vi "Input Panel Resize.vi"(8 "NewBnds":T1, 11 "Entry Panel in":refnum<vi>[](array[refnum])) -> (3 "Entry Panel out":refnum<vi>[](array[refnum]))   [LabVIEW 2015, in "CallVIStep.lvclass"]
uses:
  CallVIStep.lvclass
  <vilib>/Utility/miscctls.llb/LVRectTypeDef.ctl
  <vilib>/Utility/miscctls.llb/LVPositionTypeDef.ctl
  <vilib>/Utility/miscctls.llb/LVBoundsTypeDef.ctl
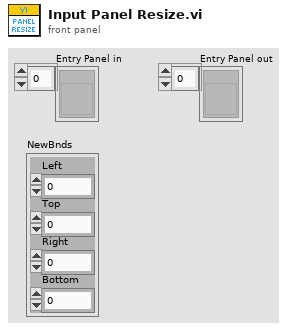
[diagram p1: front panel]
types:
  T1 = typedef "LVRectTypeDef.ctl" = cluster{"Left":i16, "Top":i16, "Right":i16, "Bottom":i16}
  T2 = typedef "LVBoundsTypeDef.ctl" = cluster{"Width":u32, "Height":u32}
  T3 = typedef "LVPositionTypeDef.ctl" = cluster{"Left":i32, "Top":i32}
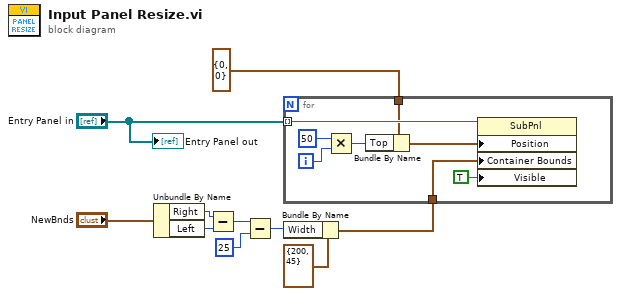
[diagram p0: block diagram]
diagram:
  n1 = Unbundle By Name("NewBnds") -> ("Right"=w7:i16, "Left"=w6:i16)
  n2 = Subtract(x=w7, y=w6) -> (x-y=w8:i16)
  n3 = Subtract(x=w8, y=i16 25) -> (x-y=w10:i16)
  n4 = Bundle By Name(cluster=T2 {"Width"=200, "Height"=45} ("Container Bounds"), "Width"=w10) -> (w2:T2)
  n5 = for {
    tunnel: "Entry Panel in" -> [w18] mode=indexing
    tunnel: T3 {"Left"=0, "Top"=0} ("Position") -> [w17]
    tunnel: w2 -> [w12]
    i -> [w14]
    n6 = Multiply(x=50, y=w14) -> (x*y=w11:i32)
    n7 = Bundle By Name(cluster=w17, "Top"=w11) -> (w16:T3)
    n8 = property class="SubPnl"(reference=w18, "Position"=w16, "Container Bounds"=w12, "Visible"=TRUE) -> ()  [unwired: 1 in, 2 out]
  }
  "Entry Panel out" <- "Entry Panel in"
